vi "HCC Open EXE Handle.vi"(1 "Status Output Locations":path[](array[path]), 2 "Connected Board ID's (Newfi)":string[](array[string]), 3 "Open Panel":T2={"Appliance Details"={"FileVersionInfo"={"FileVersion"="", "ProductName"="", "InternalName"="", "CompanyName"="", "LegalCopyright"="", "FileDescription"=""}, "Dishwasher Info"={"Open Cup Weight (gm):"=0.0, "Auto Cup Weight (gm):"=0.0, "Detergent-Dish:"="", "Inlet Temperature-Dish:"="", "Cycle Mode-Dish:"="", "Unit Control-Dish:"="", "Manufacturer-Dish:"=""}, "Washer Info"={"Hot Water Temperature (Fahrenheit):"="", "Cold Water Temperature (Fahrenheit):"="", "Capacity (cu.ft):"=0.0, "Initial Cloth Weight:"=0.0, "Cloth Lot:"=0, "Model Family:"="", "Program Name:"="", "Cycle Selection:"="", "Wash Temperature:"="", "Rinse Temperature:"="", "Load Size:"=""}, "File Name Output Array"=[], "Calibration Output Array"=[], "Appliance Common"={"Engineer:"="", "Model Number:"="", "Serial Number:"="", "Comments:"="", "Station ID:"="", "Technician:"="", "TR Number:"="", "Lab ID:"="", "Voltage:"="", "Water Pressure (PSI):"="", "Test Date:"="", "Computer Name:"="", "IP Address:"="", "Ambient RH:"="", "Frequency:"="", "Build:"="", "Filename:"="", "Test Type:"="", "Load Run #:"=0, "Ambient Temperature (F):"="", "File Path:"=path "", "Cycles Per Year"=60}, "Water Heater"={"Heating Mode:"=""}, "Dryer"={"Heat Setting:"="", "Washer Water Temperature (60 ± 5°F):"=60, "Water Hardness (PPM):"=17, "Dryness Setting:"="", "Dryer Type:"="", "Exhaust:"="", "Drying Cycle:"="", "Load Type:"="", "Nominal Load Weight"="", "Dryer Initial IMC Data"={"Measured IMC (lbs)"=7.0, "Actual Initial RMC (%)"=7.0, "RMC (Desired %)"=100.0, "Bone Dry Wt(lbs)"=7.0, "Tolerance(%)"=5.0, "Actual Final RMC (%)"=7.0, "CEF (lbf/kWh)"=0.0, "Minimum Weight (lbf)"=0.0, "Average Weight (lbf)"=0.0, "Maximum Weight (lbf)"=0.0, "Measured IMC In Range?"=FALSE, "Moisture Reduction Factor"=55.5, "Field Use Factor"=1.04, "Empty Dryer Cold Weigth"=0.0, "Energy Standard"=enum."D2-Automatic Dryer", "Weight Cloth (lbs)"=0.0, "Relative Moisture Content (%)"=0.0, "Relative Moisture Content - Avg (%)"=0.0}}}, "Display Data (RLT)"={"Status Color"=0, "Serial Number Display"="", "Cycle Count Display"=0, "Station Label Display"="", "Current Run Start Time Display"=0.0, "Board ID Display"="", "RPM Display"=0, "Current Display"=0.0, "Current Path Display"=path "", "Saving Display"=FALSE, "Unit Type Display"=enum."", "Total Time On Display"=0.0, "UI Button"=FALSE}} {"Display Data (RLT)"."Current Display" format="%.2f"; "Display Data (RLT)"."Cycle Count Display" format="%04d"; "Appliance Details"."Dryer"."Dryer Initial IMC Data"."Maximum Weight (lbf)" format="%03_6g"; "Appliance Details"."Dryer"."Dryer Initial IMC Data"."Average Weight (lbf)" format="%03_6g"; "Appliance Details"."Dryer"."Dryer Initial IMC Data"."Minimum Weight (lbf)" format="%03_6g"; "Appliance Details"."Dryer"."Dryer Initial IMC Data"."CEF (lbf/kWh)" format="%03_6g"; "Appliance Details"."Dryer"."Dryer Initial IMC Data"."Actual Final RMC (%)" format="%03_6g"; "Appliance Details"."Dryer"."Dryer Initial IMC Data"."Tolerance(%)" format="%0#_6g"; "Appliance Details"."Dryer"."Dryer Initial IMC Data"."Bone Dry Wt(lbs)" format="%03_6g"; "Appliance Details"."Dryer"."Dryer Initial IMC Data"."RMC (Desired %)" format="%0#_6g"; "Appliance Details"."Dryer"."Dryer Initial IMC Data"."Actual Initial RMC (%)" format="%03_6g"; "Appliance Details"."Dryer"."Dryer Initial IMC Data"."Measured IMC (lbs)" format="%0#_6g"}, 5 "Station Group":T1, 7 "NewVal":T2[](array[typedef]) {"Display Data (RLT)"."Current Display" format="%.2f"; "Display Data (RLT)"."Cycle Count Display" format="%04d"; "Appliance Details"."Dryer"."Dryer Initial IMC Data"."Maximum Weight (lbf)" format="%03_6g"; "Appliance Details"."Dryer"."Dryer Initial IMC Data"."Average Weight (lbf)" format="%03_6g"; "Appliance Details"."Dryer"."Dryer Initial IMC Data"."Minimum Weight (lbf)" format="%03_6g"; "Appliance Details"."Dryer"."Dryer Initial IMC Data"."CEF (lbf/kWh)" format="%03_6g"; "Appliance Details"."Dryer"."Dryer Initial IMC Data"."Actual Final RMC (%)" format="%03_6g"; "Appliance Details"."Dryer"."Dryer Initial IMC Data"."Tolerance(%)" format="%0#_6g"; "Appliance Details"."Dryer"."Dryer Initial IMC Data"."Bone Dry Wt(lbs)" format="%03_6g"; "Appliance Details"."Dryer"."Dryer Initial IMC Data"."RMC (Desired %)" format="%0#_6g"; "Appliance Details"."Dryer"."Dryer Initial IMC Data"."Actual Initial RMC (%)" format="%03_6g"; "Appliance Details"."Dryer"."Dryer Initial IMC Data"."Measured IMC (lbs)" format="%0#_6g"}, 9 "True Or False Event? (Trigger on True)":bool, 11 "error in (no error)":errorcluster, 12 "Exe Number":i32) -> (4 "Output":T2={"Appliance Details"={"FileVersionInfo"={"FileVersion"="", "ProductName"="", "InternalName"="", "CompanyName"="", "LegalCopyright"="", "FileDescription"=""}, "Dishwasher Info"={"Open Cup Weight (gm):"=0.0, "Auto Cup Weight (gm):"=0.0, "Detergent-Dish:"="", "Inlet Temperature-Dish:"="", "Cycle Mode-Dish:"="", "Unit Control-Dish:"="", "Manufacturer-Dish:"=""}, "Washer Info"={"Hot Water Temperature (Fahrenheit):"="", "Cold Water Temperature (Fahrenheit):"="", "Capacity (cu.ft):"=0.0, "Initial Cloth Weight:"=0.0, "Cloth Lot:"=0, "Model Family:"="", "Program Name:"="", "Cycle Selection:"="", "Wash Temperature:"="", "Rinse Temperature:"="", "Load Size:"=""}, "File Name Output Array"=[], "Calibration Output Array"=[], "Appliance Common"={"Engineer:"="", "Model Number:"="", "Serial Number:"="", "Comments:"="", "Station ID:"="", "Technician:"="", "TR Number:"="", "Lab ID:"="", "Voltage:"="", "Water Pressure (PSI):"="", "Test Date:"="", "Computer Name:"="", "IP Address:"="", "Ambient RH:"="", "Frequency:"="", "Build:"="", "Filename:"="", "Test Type:"="", "Load Run #:"=0, "Ambient Temperature (F):"="", "File Path:"=path "", "Cycles Per Year"=60}, "Water Heater"={"Heating Mode:"=""}, "Dryer"={"Heat Setting:"="", "Washer Water Temperature (60 ± 5°F):"=60, "Water Hardness (PPM):"=17, "Dryness Setting:"="", "Dryer Type:"="", "Exhaust:"="", "Drying Cycle:"="", "Load Type:"="", "Nominal Load Weight"="", "Dryer Initial IMC Data"={"Measured IMC (lbs)"=7.0, "Actual Initial RMC (%)"=7.0, "RMC (Desired %)"=100.0, "Bone Dry Wt(lbs)"=7.0, "Tolerance(%)"=5.0, "Actual Final RMC (%)"=7.0, "CEF (lbf/kWh)"=0.0, "Minimum Weight (lbf)"=0.0, "Average Weight (lbf)"=0.0, "Maximum Weight (lbf)"=0.0, "Measured IMC In Range?"=FALSE, "Moisture Reduction Factor"=55.5, "Field Use Factor"=1.04, "Empty Dryer Cold Weigth"=0.0, "Energy Standard"=enum."D2-Automatic Dryer", "Weight Cloth (lbs)"=0.0, "Relative Moisture Content (%)"=0.0, "Relative Moisture Content - Avg (%)"=0.0}}}, "Display Data (RLT)"={"Status Color"=0, "Serial Number Display"="", "Cycle Count Display"=0, "Station Label Display"="", "Current Run Start Time Display"=0.0, "Board ID Display"="", "RPM Display"=0, "Current Display"=0.0, "Current Path Display"=path "", "Saving Display"=FALSE, "Unit Type Display"=enum."", "Total Time On Display"=0.0, "UI Button"=FALSE}} {"Display Data (RLT)"."Current Display" format="%.2f"; "Display Data (RLT)"."Cycle Count Display" format="%04d"; "Appliance Details"."Dryer"."Dryer Initial IMC Data"."Maximum Weight (lbf)" format="%03_6g"; "Appliance Details"."Dryer"."Dryer Initial IMC Data"."Average Weight (lbf)" format="%03_6g"; "Appliance Details"."Dryer"."Dryer Initial IMC Data"."Minimum Weight (lbf)" format="%03_6g"; "Appliance Details"."Dryer"."Dryer Initial IMC Data"."CEF (lbf/kWh)" format="%03_6g"; "Appliance Details"."Dryer"."Dryer Initial IMC Data"."Actual Final RMC (%)" format="%03_6g"; "Appliance Details"."Dryer"."Dryer Initial IMC Data"."Tolerance(%)" format="%0#_6g"; "Appliance Details"."Dryer"."Dryer Initial IMC Data"."Bone Dry Wt(lbs)" format="%03_6g"; "Appliance Details"."Dryer"."Dryer Initial IMC Data"."RMC (Desired %)" format="%0#_6g"; "Appliance Details"."Dryer"."Dryer Initial IMC Data"."Actual Initial RMC (%)" format="%03_6g"; "Appliance Details"."Dryer"."Dryer Initial IMC Data"."Measured IMC (lbs)" format="%0#_6g"}, 15 "error out":errorcluster)   [LabVIEW 2018]
uses:
  Utility/Save File/Public/Type Definitions/Save File Washer.ctl
  Utility/Save File/File Setup (Public)/Type Definition/Save File DISH Dishwasher Details.ctl
  <vilib>/Platform/fileVersionInfo.llb/FileVersionInformation.ctl
  Washer DOE/Type Definitions/DOE Appliance Common.ctl
  Utility/Custom Pallet Controls/Custom Pallet String.ctl
  Utility/Save File/File Setup (Public)/Type Definition/DPT IMC Data.ctl
  Washer DOE/Type Definitions/DOE Dryer Standard.ctl
  Utility/Save File/Public/Type Definitions/Save File Appliance Display.ctl
  Utility/Save File/Public/Type Definitions/Save File Unit Type.ctl
  Type Definitions/HCC Station Group.ctl
  Utility/Save File/Save File.lvlib
  Utility/Save File/File Setup.lvlib
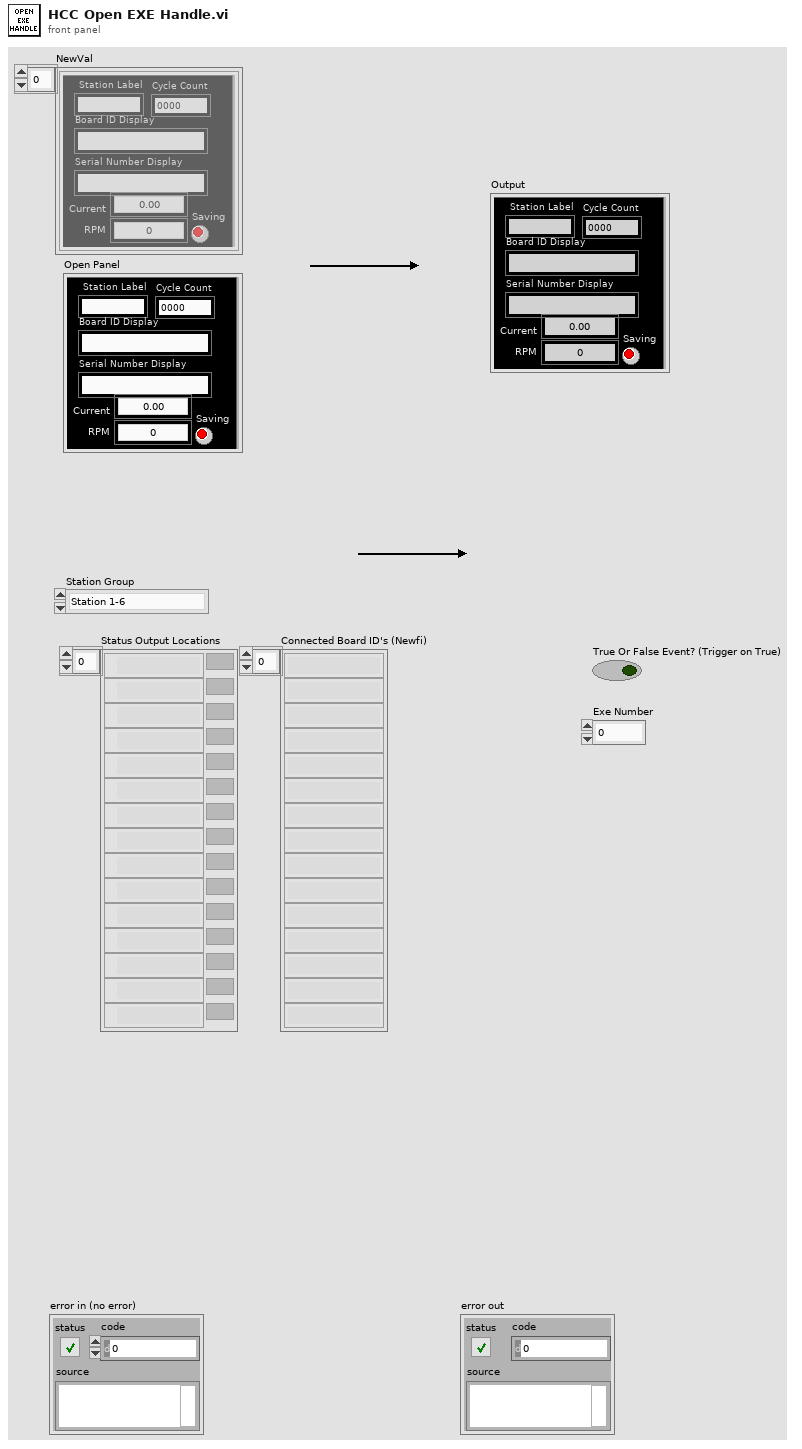
[diagram p1: front panel]
types:
  T1 = typedef "HCC Station Group.ctl" = enum16{"Station 1-6", "Station 7-12", "Station 13-18", "Station 19-24"}
  T2 = typedef "Save File.lvlib/Save File Washer.ctl" = cluster{"Appliance Details":T3, "Display Data (RLT)":T9}
  T3 = typedef "File Setup.lvlib/Save File DISH Dishwasher Details.ctl" = cluster{"FileVersionInfo":T4, "Dishwasher Info":cluster{"Open Cup Weight (gm):":dbl, "Auto Cup Weight (gm):":dbl, "Detergent-Dish:":string, "Inlet Temperature-Dish:":string, "Cycle Mode-Dish:":string, "Unit Control-Dish:":string, "Manufacturer-Dish:":string}, "Washer Info":cluster{"Hot Water Temperature (Fahrenheit):":string, "Cold Water Temperature (Fahrenheit):":string, "Capacity (cu.ft):":dbl, "Initial Cloth Weight:":dbl, "Cloth Lot:":i32, "Model Family:":string, "Program Name:":string, "Cycle Selection:":string, "Wash Temperature:":string, "Rinse Temperature:":string, "Load Size:":string}, "File Name Output Array":string[][], "Calibration Output Array":string[][], "Appliance Common":T5, "Water Heater":cluster{"Heating Mode:":string}, "Dryer":cluster{"Heat Setting:":T6, "Washer Water Temperature (60 ± 5°F):":u16, "Water Hardness (PPM):":u16, "Dryness Setting:":T6, "Dryer Type:":string, "Exhaust:":string, "Drying Cycle:":string, "Load Type:":string, "Nominal Load Weight":string, "Dryer Initial IMC Data":T7}}
  T4 = typedef "FileVersionInformation.ctl" = cluster{"FileVersion":string, "ProductName":string, "InternalName":string, "CompanyName":string, "LegalCopyright":string, "FileDescription":string}
  T5 = typedef "DOE Appliance Common.ctl" = cluster{"Engineer:":string, "Model Number:":string, "Serial Number:":string, "Comments:":string, "Station ID:":string, "Technician:":string, "TR Number:":string, "Lab ID:":string, "Voltage:":string, "Water Pressure (PSI):":string, "Test Date:":string, "Computer Name:":string, "IP Address:":string, "Ambient RH:":string, "Frequency:":string, "Build:":string, "Filename:":string, "Test Type:":string, "Load Run #:":i32, "Ambient Temperature (F):":string, "File Path:":path, "Cycles Per Year":u32}
  T6 = typedef "Custom Pallet String.ctl" = string
  T7 = typedef "DPT IMC Data.ctl" = cluster{"Measured IMC (lbs)":dbl, "Actual Initial RMC (%)":dbl, "RMC (Desired %)":dbl, "Bone Dry Wt(lbs)":dbl, "Tolerance(%)":dbl, "Actual Final RMC (%)":dbl, "CEF (lbf/kWh)":dbl, "Minimum Weight (lbf)":dbl, "Average Weight (lbf)":dbl, "Maximum Weight (lbf)":dbl, "Measured IMC In Range?":bool, "Moisture Reduction Factor":dbl, "Field Use Factor":dbl, "Empty Dryer Cold Weigth":dbl, "Energy Standard":T8, "Weight Cloth (lbs)":dbl, "Relative Moisture Content (%)":dbl, "Relative Moisture Content - Avg (%)":dbl}
  T8 = typedef "DOE Dryer Standard.ctl" = enum16{"D2-Automatic Dryer", "D2-Timer Dryer", "D1-Automatic Dryer", "D1-Timer Dryer", "Other"}
  T9 = typedef "Save File Appliance Display.ctl" = cluster{"Status Color":u32, "Serial Number Display":string, "Cycle Count Display":i32, "Station Label Display":string, "Current Run Start Time Display":dbl, "Board ID Display":string, "RPM Display":u32, "Current Display":dbl, "Current Path Display":path, "Saving Display":bool, "Unit Type Display":T10, "Total Time On Display":dbl, "UI Button":bool}
  T10 = typedef "Save File.lvlib/Save File Unit Type.ctl" = enum32{"", "Viper", "Hawk", "2015"}
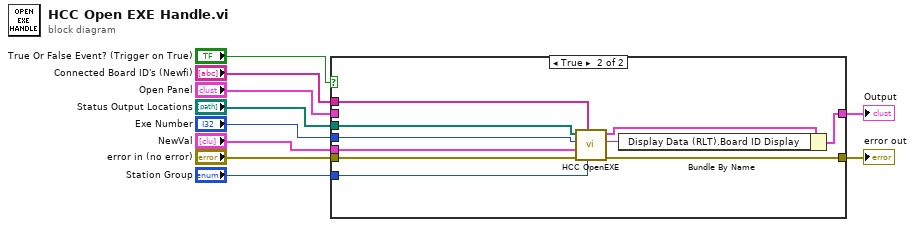
[diagram p0: block diagram]
diagram:
  n1 = case shown="True" "True Or False Event? (Trigger on True)" {
    tunnel: [w12 w22] -> w3
    tunnel: "Open Panel" -> [w12 _]
    tunnel: [w11 w21] -> w5
    tunnel: "Connected Board ID's (Newfi)" -> [_ w20]
    tunnel: "Status Output Locations" -> [_ w19]
    tunnel: "Exe Number" -> [_ w18]
    tunnel: "error in (no error)" -> [w11 w13]
    tunnel: "NewVal" -> [_ w17]
    tunnel: "Station Group" -> [_ w14]
    frame False {
      # "When the button is depressed. It runs the event\ntwice..this causes issues calling the search process.\nThis case structure filters only the true event"
    }
    frame True {
      n2 = call "HCC OpenEXE.vi"("Station Group"=w14, "Connected Board ID's (Newfi)"=w20, "error in (no error)"=w13, "NewVal"=w17, "Exe Number (1-24)"=w18, "Status Output Locations"=w19) -> ("error out"=w21:errorcluster, "Board ID"=w15:string, "Dryer"=w16:T2)  [unwired: 3 in]
      n3 = Bundle By Name(cluster=w16, "Display Data (RLT).Board ID Display"=w15) -> (w22:T2)
    }
  }
  "error out" <- w5
  "Output" <- w3
